vi "waypointQdone.vi"(9 "Waypoint Queue":refnum<queue>, 10 "missions queue":refnum<queue>, 11 "Old Missions":refnum<class "GenericMission.lvclass">[](array[class])) -> (2 "new mission?":bool, 3 "Old Missions (updated)":refnum<class "GenericMission.lvclass">[](array[class]))   [LabVIEW 2013]
doc: "When there's one mission left in the queue, the mission has been compleated. This vi checks to see if the mission is compleated, removes the compleated mission from the queue, and adds it to the compleated missions array."
uses:
  Logic/Classes/Waypoint/Waypoint.lvclass
  Logic/Classes/Missions/GenericMission/GenericMission.lvclass
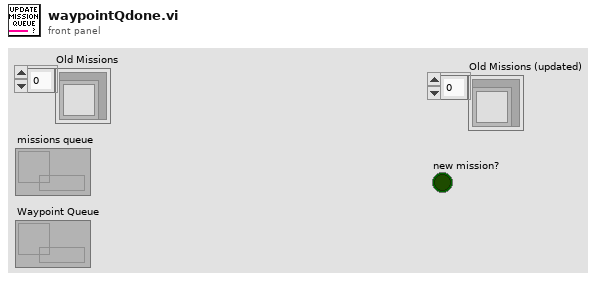
[diagram p1: front panel]
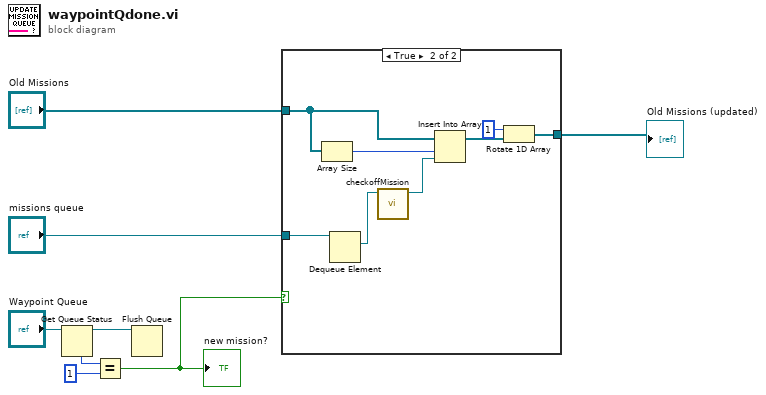
[diagram p0: block diagram]
diagram:
  n1 = Get Queue Status(queue="Waypoint Queue") -> (queue out=w1:refnum<queue>, # elements in queue=w8:i32)  [unwired: 2 in, 6 out]
  n2 = Equal?(x=w8, y=1) -> (x = y?=w6:bool)
  "new mission?" <- w6
  n3 = Flush Queue(queue=w1) -> ()  [unwired: 1 in, 3 out]
  n4 = case shown="True" w6 {
    tunnel: "missions queue" -> [_ w17]
    tunnel: "Old Missions" -> [w9 w15]
    tunnel: [w9 w12] -> w3
    frame False {
    }
    frame True {
      n5 = Array Size(array=w15) -> (size(s)=w14:i32)
      n6 = Dequeue Element(queue=w17) -> (element=w11:refnum<class "GenericMission.lvclass">)  [unwired: 2 in, 3 out]
      n7 = call "checkoffMission.vi"("GenericMission in"=w11) -> ("GenericMission out"=w10:refnum<class "GenericMission.lvclass">)  [unwired: 9 in, 1 out]
      n8 = Insert Into Array(array=w15, index=w14, new element=w10) -> (w16:refnum<class "GenericMission.lvclass">[])
      n9 = Rotate 1D Array(1:w16, 2:1 ("n")) -> (0:w12:refnum<class "GenericMission.lvclass">[])
    }
  }
  "Old Missions (updated)" <- w3
